vi "Configure TV Trigger Line Number [TV] Core.vi"(8 "error in (no error)":errorcluster, 10 "tv line number (1)":i32=1, 11 "IVI_Scope in":refnum<class "IVI_Scope.lvclass">) -> (0 "error out":errorcluster, 3 "IVI_Scope out":refnum<class "IVI_Scope.lvclass">)   [LabVIEW 2016, in "IVI_Scope.lvlib" / "IVI_Scope.lvclass"]
doc: "This VI configures the TV line upon which the oscilloscope triggers. The line number is absolute and not relative to the field of the TV signal.\n\nNote\n\n(1) This VI affects instrument behavior only if the trigger type is set to\n IVISCOPE_VAL_TV_TRIGGER and the TV trigger event is set to\n IVISCOPE_VAL_TV_EVENT_LINE_NUMBER. Call the IviScope\n Configure Trigger and the IviScope Configure TV Trigger Source [TV]\n VIs to set the trigger type and TV trigger event before calling this VI\n.\n(2) This VI is part of the IviScopeTVTrigger [TV] extension group."
uses:
  IVI_Scope.lvclass
  IVI_Scope.lvclass/IVI_Scope.ctl
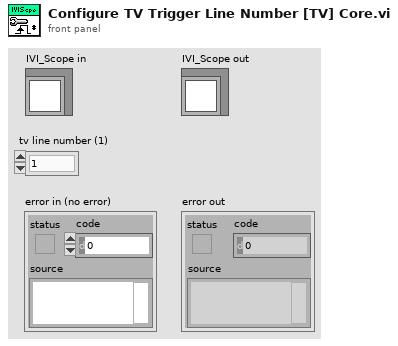
[diagram p1: front panel]
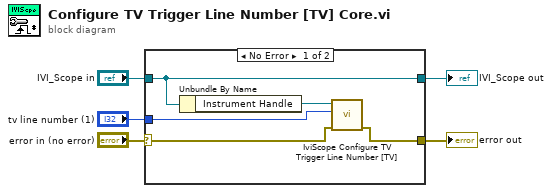
[diagram p0: block diagram]
diagram:
  n1 = case shown="No Error" "error in (no error)" {
    selector: "error in (no error)" -> [w8 w12]
    tunnel: [w7 w12] -> w4
    tunnel: [w10 w11] -> w2
    tunnel: "IVI_Scope in" -> [w10 w11]
    tunnel: "tv line number (1)" -> [w6 _]
    frame No Error {
      n2 = Unbundle By Name(w10) -> ("Instrument Handle"=w9:refnum<k15>)
      n3 = call <vilib>:"IviScope Configure TV Trigger Line Number [TV].vi"("error in (no error)"=w8, "tv line number (1)"=w6, "instrument handle"=w9) -> ("error out"=w7:errorcluster)  [unwired: 7 in, 1 out]
    }
    frame Error {
    }
  }
  "error out" <- w4
  "IVI_Scope out" <- w2
